vi "SpinnyGlo.vi"() -> ()   [LabVIEW 2014]
uses:
  <vilib>/userdefined/High Color/IMAQdx.ctl
  <vilib>/LabVIEW Interface for Arduino/LabVIEW Interface for Arduino.lvlib
  <vilib>/vision/driver/NI_Vision_Acquisition_Software.lvlib
panel:
  out "Steps per Image":dbl
  out "Total Steps":dbl
  out "Images Acquired":i32
  in  "File Name":string
  in  "Save Location":path
  out "Image":T1(plugin-control)
  out "Degrees per Step":dbl
  out "Degrees per Image":dbl
  in  "Number of Images":dbl
  in  "Camera Name":T2
  out "Steps\nRemaining":u32
  in  "Angular Increment":dbl
  in  "Exit":bool
  in  "Home":bool
  in  "Stop":bool
  in  "MoveToGo":bool
  in  "MoveForGo":bool
  in  "Direction":bool
  out "Current Position":dbl format="%#.2f"
  in  "Move For (+/-360 max)":dbl
  in  "Move To":dbl
  # "CW"
  # "CCW"
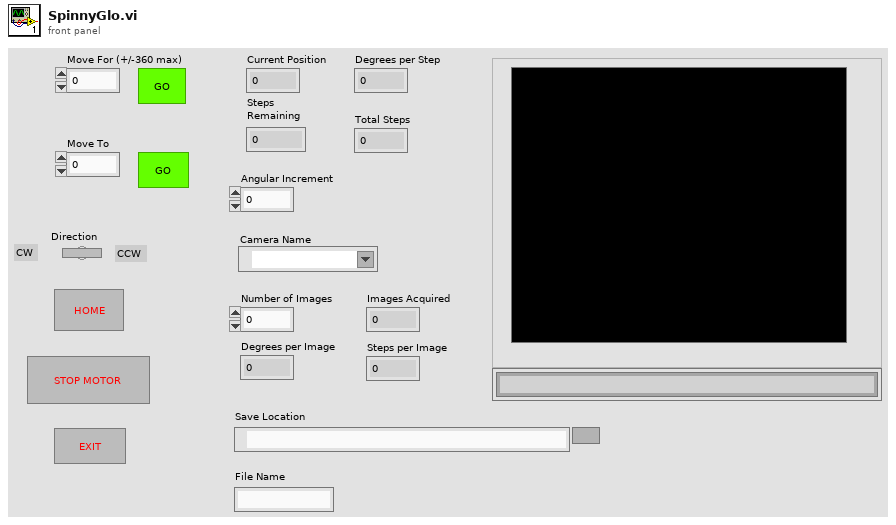
[diagram p1: front panel]
types:
  T1 = typedef "IMAQ Image.ctl" = refnum<image>
  T2 = typedef "IMAQdx.ctl" = refnum<k21>
  T3 = enum16{"Enabled", "Disabled", "Disabled and Grayed Out"}
  T4 = enum8{"Enabled", "Disabled", "Disabled and Grayed Out"}
  T5 = typedef "LabVIEW Interface for Arduino.lvlib/Arduino Resource.ctl" = cluster{"VISA resource":refnum<visa-resource-name>, "Board Type":T6, "Connection Type":enum8{"USB / Serial"}, "Bytes Per Packet (15)":u8}
  T6 = typedef "LabVIEW Interface for Arduino.lvlib/Board Type.ctl" = enum16{"Uno", "Dimuelanove w/Atmega 328", "Mega 2560"}
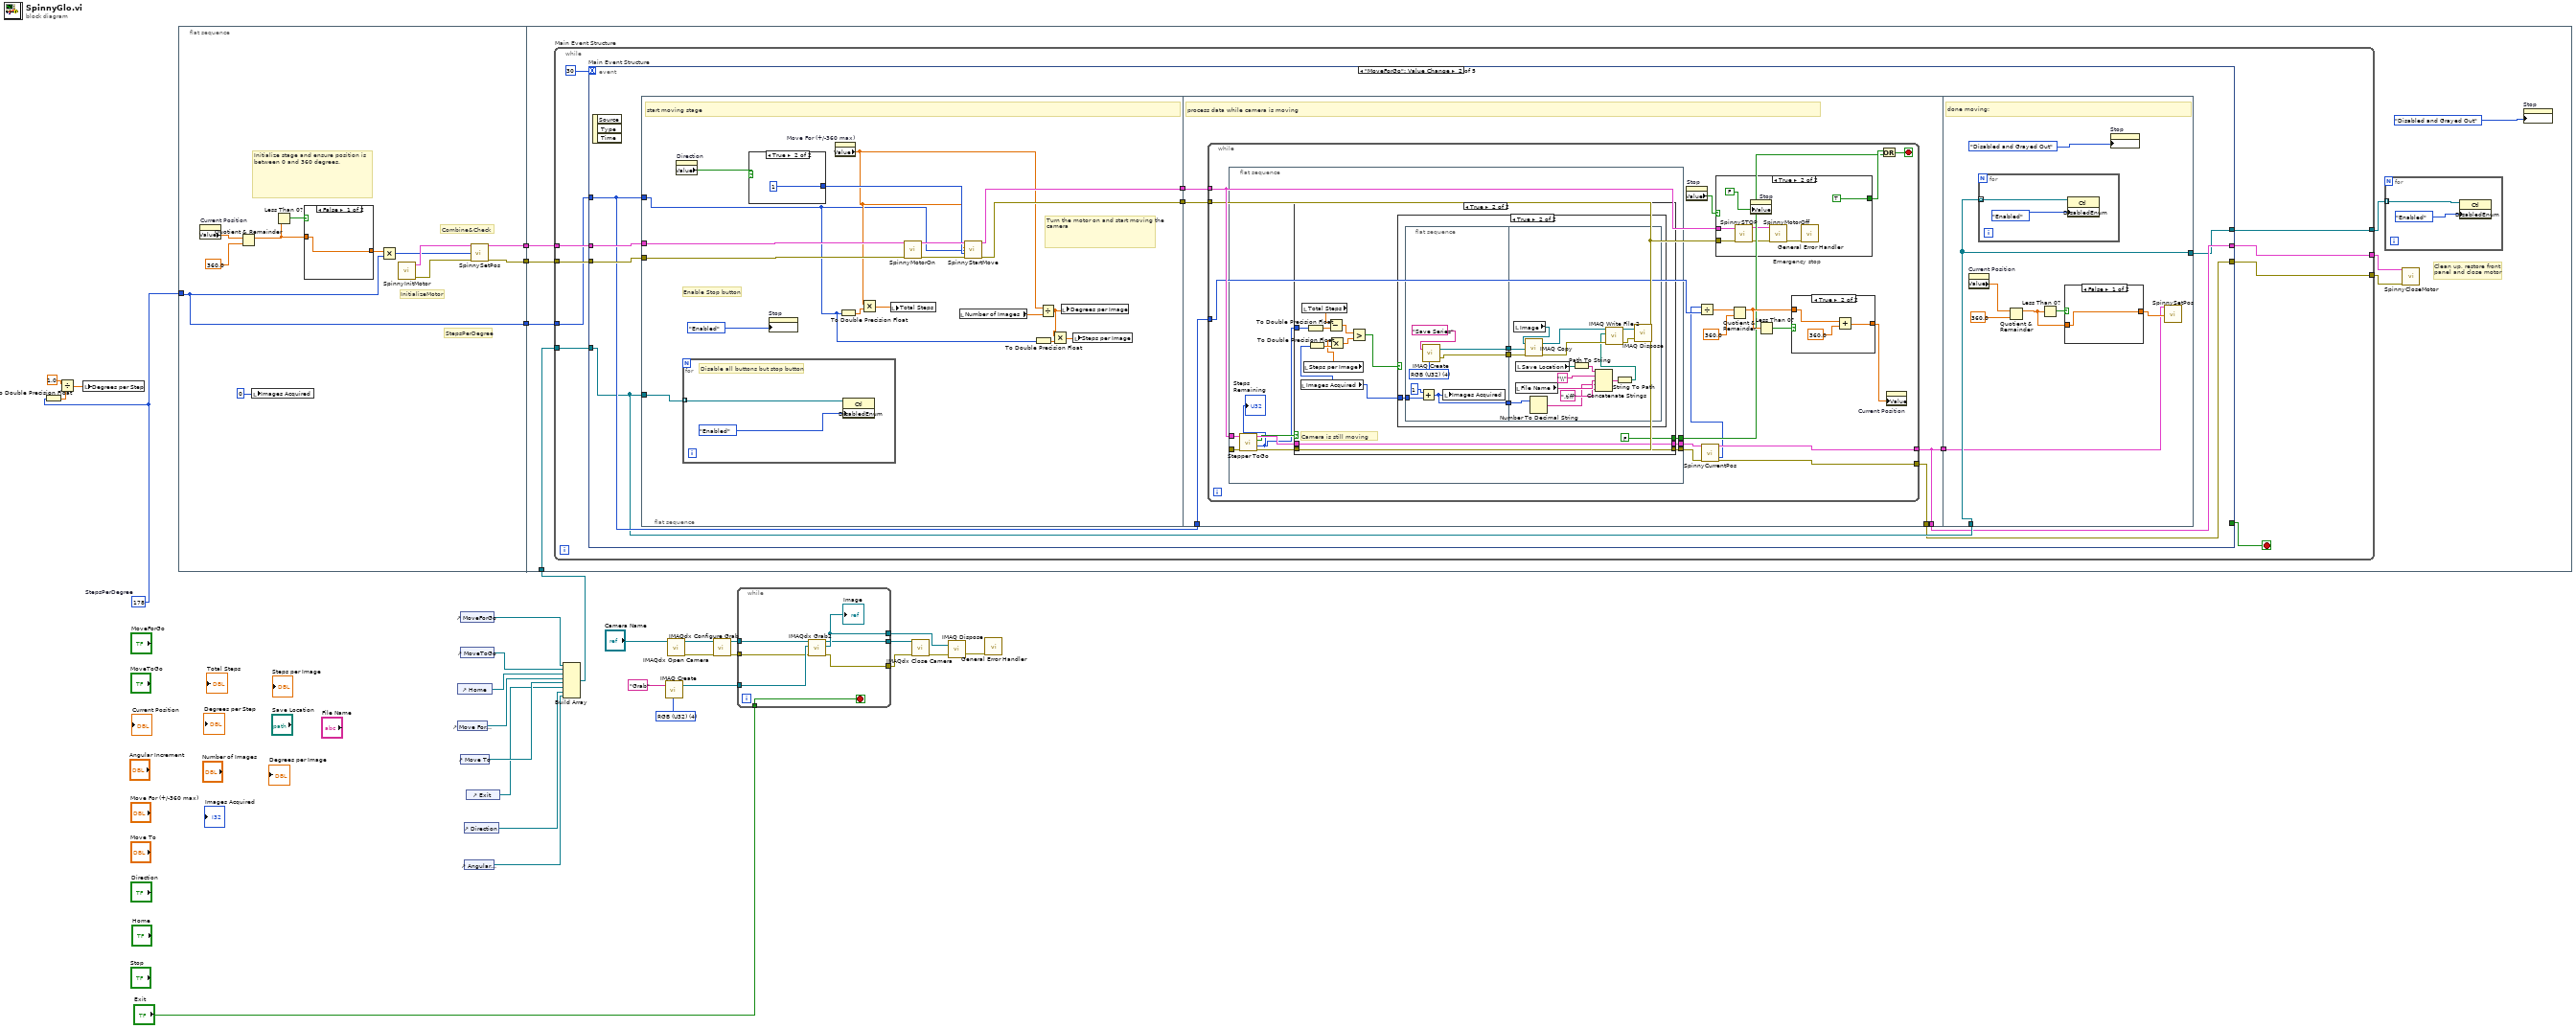
[diagram p0: block diagram]
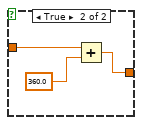
[diagram p2: hidden frame]
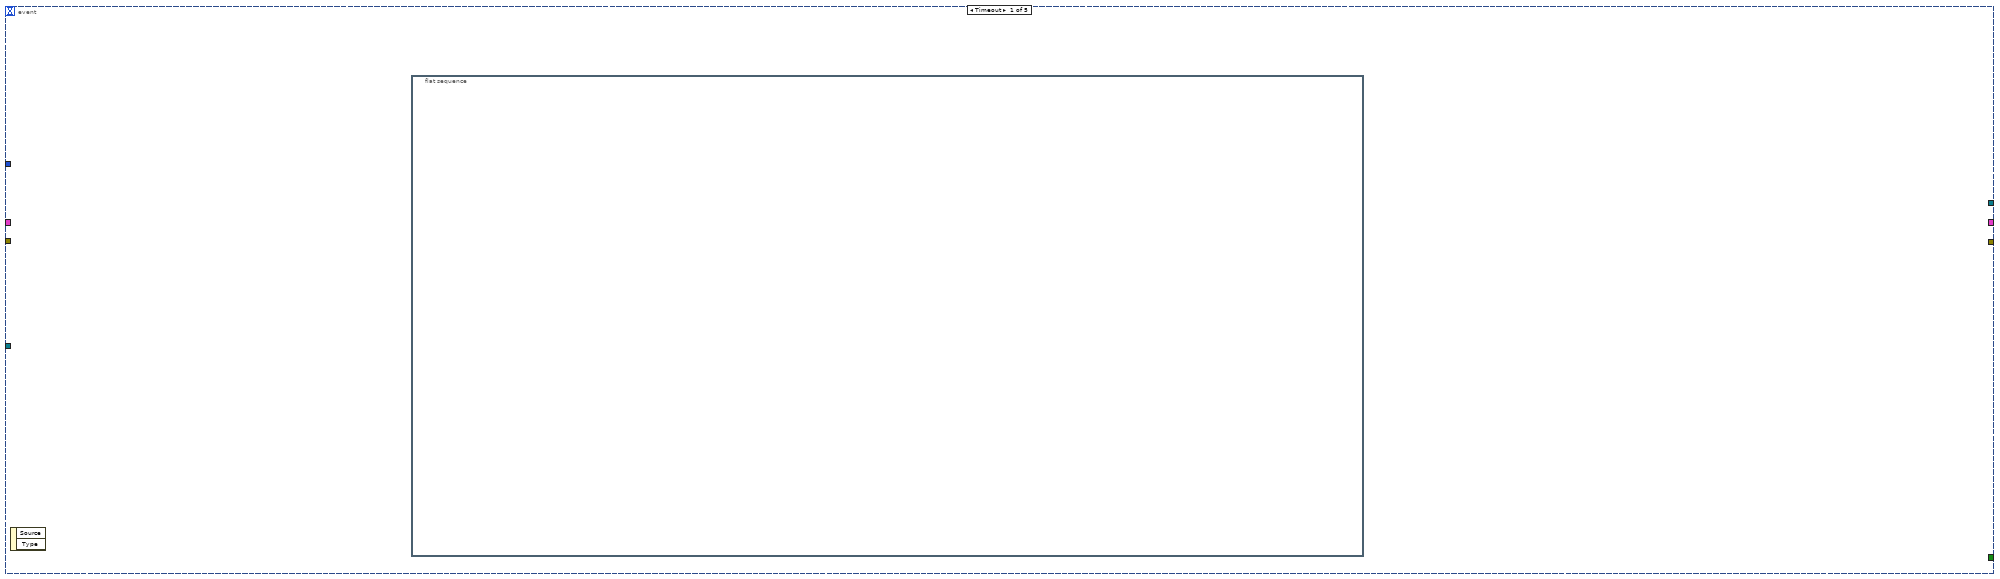
[diagram p3: hidden frame]
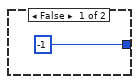
[diagram p4: hidden frame]
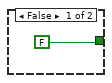
[diagram p6: hidden frame]
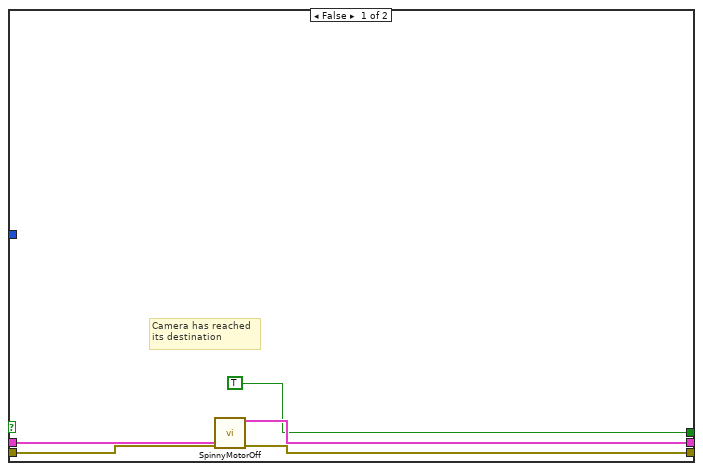
[diagram p7: hidden frame]
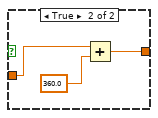
[diagram p9: hidden frame]
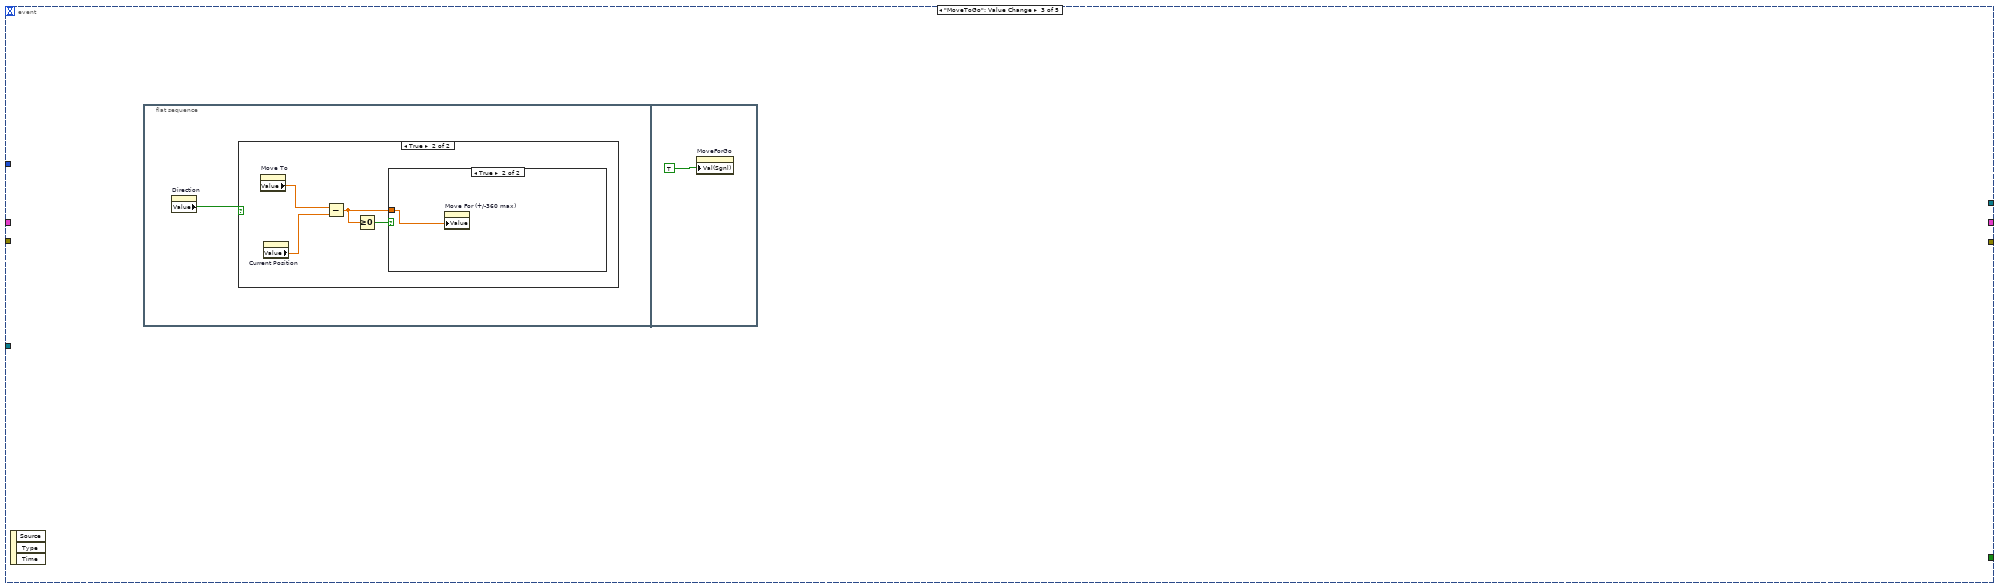
[diagram p10: hidden frame]
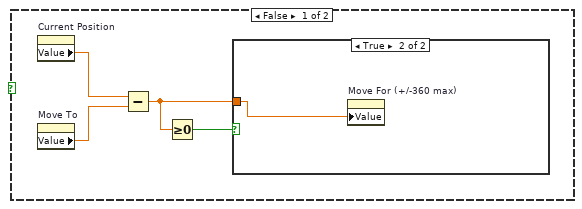
[diagram p11: hidden frame]
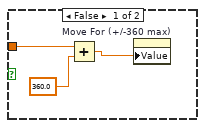
[diagram p12: hidden frame]
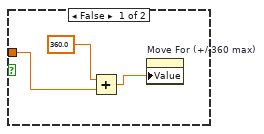
[diagram p13: hidden frame]
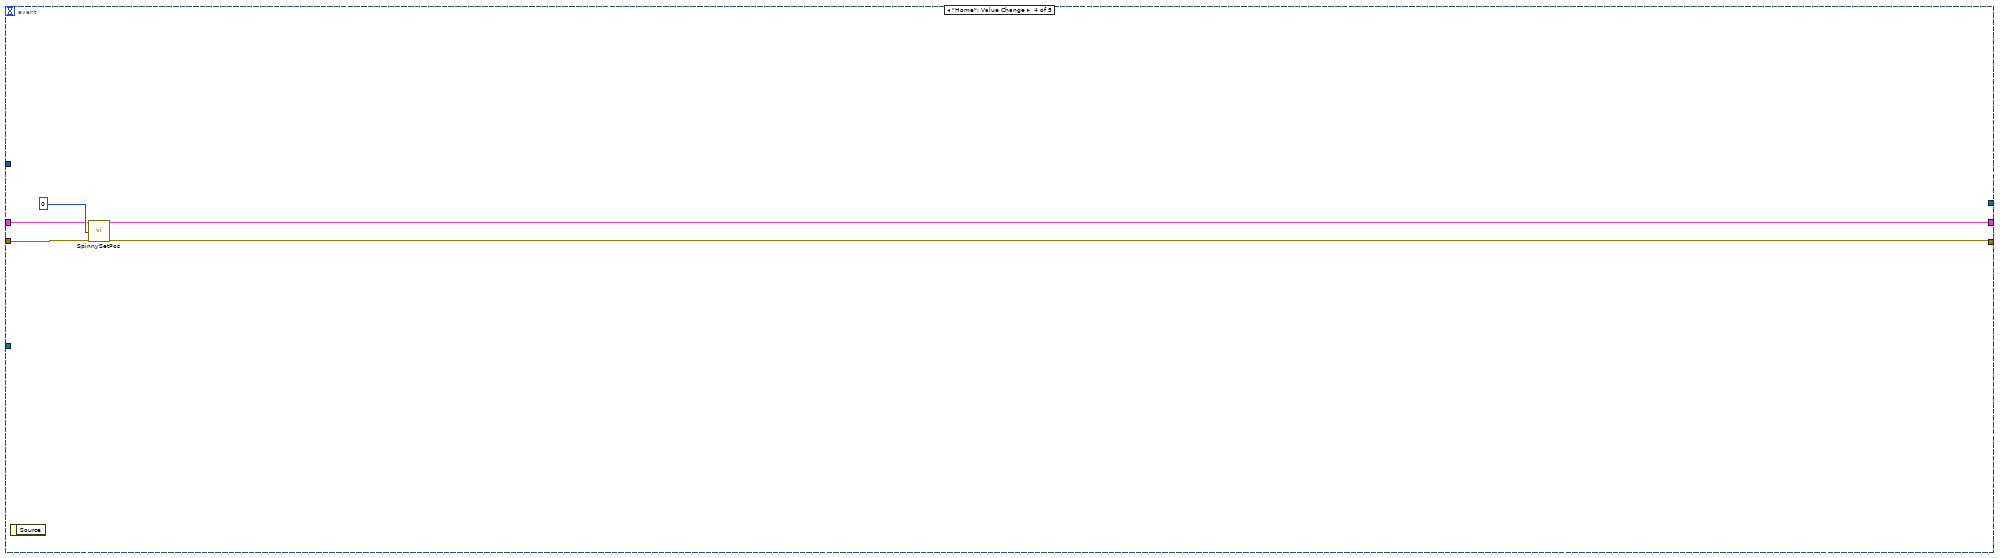
[diagram p14: hidden frame]
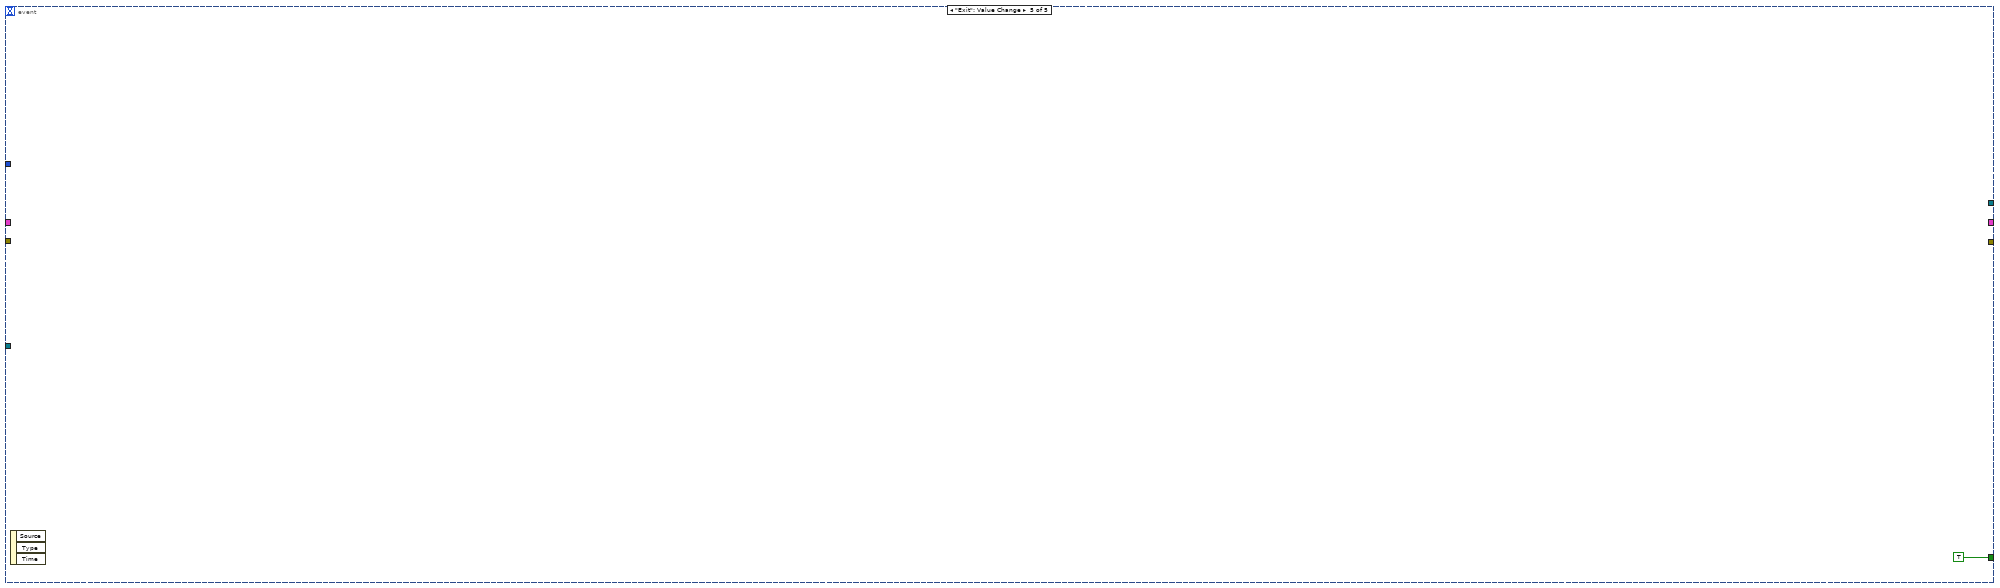
[diagram p15: hidden frame]
diagram:
  w18 = u32 4 items=["Grayscale (U8)", "Grayscale (I16)", "Grayscale (SGL)", "Complex (CSG)", "RGB (U32)", "HSL (U32)", "RGB (U64)", "Grayscale (U16)", ""] ("Image Type")
  w2 = 178  # StepsPerDegree
  n1 = To Double Precision Float(number=w2) -> (double precision float=w5:dbl)
  n2 = Divide(x=1.0, y=w5) -> (x/y=w3:dbl)
  n3 = local write "Degrees per Step"(w3) -> ()
  n4 = flat-sequence {
    tunnel: w2 -> [w32]
    tunnel: [w34] -> w30
    tunnel: [w33] -> w29
    tunnel: [w32] -> w19
    tunnel: w30 -> [w53]
    tunnel: w29 -> [w52]
    tunnel: w20 -> [w54]
    tunnel: w19 -> [w51]
    frame #0 {
      # "StepsPerDegree"
      # "Combine&Check"
      # "InitializeMotor"
      # "Initialize stage and ensure position is between 0 and 360 degrees."
      n5 = property on="Current Position" class="DigNum (strict)"() -> ("Value"=w42:dbl)  [unwired: 2 in, 2 out]
      n6 = Quotient & Remainder(x=w42, y=sgl 360.0) -> (x-y*floor(x/y)=w39:dbl)  [unwired: 1 out]
      n7 = local write "Images Acquired"(0) -> ()
      n8 = Less Than 0?(x=w39) -> (x < 0?=w40:bool)
      n9 = case shown="False" w40 {
        tunnel: w39 -> [w43 w46]
        tunnel: [w43 w44] -> w38
        frame False {
        }
        frame True {
          n10 = Add(x=w46, y=sgl 360.0) -> (x+y=w44:dbl)
        }
      }
      n11 = Multiply(x=w38, y=w32) -> (x*y=w35:i32)
      n12 = call "SpinnyInitMotor.vi"() -> ("error out"=w36:errorcluster, "Arduino Resource Out"=w37:T5)  [unwired: 10 in]
      n13 = call "SpinnySetPos.vi"("Arduino Resource"=w37, "position"=w35, "error in"=w36) -> ("Arduino Resource Out"=w34:T5, "error out"=w33:errorcluster)  [unwired: 15 in]
    }
    frame #1 {
      # "Clean up, restore front\npanel and close motor"
      n14 = while "Main Event Structure" {
        tunnel: w54 -> [w64]
        tunnel: w53 -> [w63]
        tunnel: w52 -> [w62]
        tunnel: w51 -> [w61]
        tunnel: [w60] -> w48
        tunnel: [w59] -> w50
        tunnel: [w58] -> w49
        stop <- w57 stop-if-true
        n15 = event "Main Event Structure" shown="[1] \"MoveForGo\": Value Change" {
          selector: _ -> [_ _ _ _ _]
          dyn-events: _ -> [_ _ _ _ _]
          timeout: 30 -> [_ _ _ _ _]
          tunnel: w64 -> [_ w69 _ _ _]
          tunnel: w63 -> [_ w75 _ w220 _]
          tunnel: w62 -> [_ w74 _ w219 _]
          tunnel: w61 -> [_ w71 _ _ _]
          tunnel: [_ w68 _ w218 _] -> w59
          tunnel: [_ w67 _ w217 _] -> w58
          tunnel: [_ w66 _ _ _] -> w60
          tunnel: [_ _ _ _ TRUE] -> w57
          event Timeout {
            n16 = event-data() -> ()  [unwired: 1 in, 2 out]
            n17 = flat-sequence {
              frame #0 {
              }
            }
          }
          event "MoveForGo": Value Change {
            n18 = event-data() -> ()  [unwired: 1 in, 3 out]
            n19 = flat-sequence {
              tunnel: w69 -> [w93]
              tunnel: w75 -> [w90]
              tunnel: w74 -> [w88]
              tunnel: w71 -> [w79]
              tunnel: [w85] -> w73
              tunnel: [w84] -> w72
              tunnel: w73 -> [w102]
              tunnel: w72 -> [w101]
              tunnel: w71 -> [w100]
              tunnel: [w99] -> w70
              tunnel: [w99] -> w68
              tunnel: [w98] -> w67
              tunnel: w70 -> [w185]
              tunnel: w69 -> [w186]
              tunnel: [w186] -> w66
              frame #0 {
                # "Turn the motor on and start moving the camera"
                # "start moving stage"
                # "Enable Stop button"
                n20 = property on="Direction" class="Bool (strict)"() -> ("Value"=w91:bool)  [unwired: 2 in, 2 out]
                n21 = for {
                  tunnel: w93 -> [w97] mode=indexing
                  # "Disable all buttons but stop button"
                  n22 = property class="Ctl"(reference=w97, "DisabledEnum"=T3."Enabled") -> ()  [unwired: 1 in, 2 out]
                }
                n23 = case shown="True" w91 {
                  tunnel: [-1 1] -> w86
                  frame False {
                  }
                  frame True {
                  }
                }
                n24 = property on="Stop" class="Bool (strict)"("DisabledEnum"=T4."Enabled") -> ()  [unwired: 2 in, 2 out]
                n25 = property on="Move For (+/-360 max)" class="DigNum (strict)"() -> ("Value"=w81:dbl)  [unwired: 2 in, 2 out]
                n26 = To Double Precision Float(number=w79) -> (double precision float=w82:dbl)
                n27 = Multiply(x=w81, y=w82) -> (x*y=w80:dbl)
                n28 = local write "Total Steps"(w80) -> ()
                n29 = call "SpinnyMotorOn.vi"("Arduino Resource"=w90, "error in"=w88) -> ("Arduino Resource Out"=w89:T5, "error out"=w87:errorcluster)  [unwired: 12 in]
                n30 = local read "Number of Images"() -> (w83:dbl)
                n31 = call "SpinnyStartMove.vi"("Arduino Resource"=w89, "Degrees To Move"=w81, "Steps Per Degree"=w79, "Direction"=w86, "error in"=w87) -> ("Arduino Resource Out"=w85:T5, "error out"=w84:errorcluster)  [unwired: 9 in]
                n32 = To Double Precision Float(number=w79) -> (double precision float=w78:dbl)
                n33 = Divide(x=w81, y=w83) -> (x/y=w77:dbl)
                n34 = Multiply(x=w77, y=w78) -> (x*y=w76:dbl)
                n35 = local write "Degrees per Image"(w77) -> ()
                n36 = local write "Steps per Image"(w76) -> ()
              }
              frame #1 {
                # "process data while camera is moving"
                n37 = while {
                  tunnel: w102 -> [w117]
                  tunnel: w101 -> [w116]
                  tunnel: [w115] -> w98
                  tunnel: [w113] -> w99
                  tunnel: w100 -> [w112]
                  stop <- w105 stop-if-true
                  n38 = flat-sequence {
                    tunnel: w116 -> [w140]
                    tunnel: w117 -> [w139]
                    tunnel: [w135] -> w118
                    tunnel: [w134] -> w119
                    tunnel: [w133] -> w106
                    frame #0 {
                      n39 = call <vilib>:"Stepper ToGo.vi"("error in"=w140, "Arduino Resource"=w139) -> ("error out"=w137:errorcluster, "Steps remaining"=w132:u32, "Steps Remaining?"=w136:bool, "Arduino Resource Out"=w138:T5)  [unwired: 6 in]
                      "Steps\nRemaining" <- w132
                      n40 = case shown="True" w136 {
                        tunnel: w138 -> [w145 w157]
                        tunnel: w137 -> [w144 w156]
                        tunnel: [w143 w157] -> w134
                        tunnel: [w142 w156] -> w135
                        tunnel: [TRUE FALSE] -> w133
                        tunnel: w132 -> [_ w154]
                        frame False {
                          # "Camera has reached\nits destination"
                          n41 = call "SpinnyMotorOff.vi"("Arduino Resource"=w145, "error in"=w144) -> ("Arduino Resource Out"=w143:T5, "error out"=w142:errorcluster)  [unwired: 12 in]
                        }
                        frame True {
                          # "Camera is still moving"
                          n42 = local read "Images Acquired"() -> (w148:i32)
                          n43 = local read "Total Steps"() -> (w152:dbl)
                          n44 = local read "Steps per Image"() -> (w147:dbl)
                          n45 = To Double Precision Float(number=w154) -> (double precision float=w153:dbl)
                          n46 = To Double Precision Float(number=w148) -> (double precision float=w149:dbl)
                          n47 = Subtract(x=w152, y=w153) -> (x-y=w151:dbl)
                          n48 = Multiply(x=w147, y=w149) -> (x*y=w146:dbl)
                          n49 = Greater?(x=w151, y=w146) -> (0:w150:bool)
                          n50 = case shown="True" w150 {
                            tunnel: w148 -> [_ w159]
                            frame False {
                            }
                            frame True {
                              n51 = flat-sequence {
                                tunnel: [w166] -> w161
                                tunnel: [w165] -> w160
                                tunnel: w159 -> [w164]
                                tunnel: [w162] -> w158
                                tunnel: w161 -> [w183]
                                tunnel: w160 -> [w179]
                                tunnel: w158 -> [w172]
                                frame #0 {
                                w167 = u16 4 items=["Grayscale (U8)", "Grayscale (I16)", "Grayscale (SGL)", "Complex (CSG)", "RGB (U32)", "HSL (U32)", "RGB (U64)", "Grayscale (U16)", ""]
                                n52 = Add(x=1, y=w164) -> (x+y=w162:i32)
                                n53 = call "IMAQ Create"("Image Name"="Save Series", "Image Type"=w167) -> ("New Image"=w166:T1, "error out"=w165:errorcluster)  [unwired: 3 in]
                                n54 = local write "Images Acquired"(w162) -> ()
                                }
                                frame #1 {
                                n55 = local read "Image"() -> (w184:T1)
                                n56 = local read "File Name"() -> (w174:string)
                                n57 = local read "Save Location"() -> (w176:path)
                                n58 = call "IMAQ Copy"("error in (no error)"=w179, "Image Dst"=w183, "Image Src"=w184) -> ("error out"=w178:errorcluster, "Image Dst Out"=w182:T1)  [unwired: 3 in]
                                n59 = Number To Decimal String(number=w172) -> (decimal integer string=w171:string)  [unwired: 1 in]
                                n60 = Path To String(path=w176) -> (string=w177:string)
                                n61 = Concatenate Strings(w177, "\\", w174, w171, ".tiff") -> (w170:string)
                                n62 = String To Path(string=w170) -> (path=w169:path)
                                n63 = call-poly "IMAQ Write File 2"("error in (no error)"=w178, "File Path"=w169, "Image"=w182) -> ("error out"=w180:errorcluster, "Image Out (duplicate)"=w181:T1)  [unwired: 7 in]
                                n64 = call "IMAQ Dispose"("Image"=w181, "error in (no error)"=w180) -> ()  [unwired: 4 in, 1 out]
                                }
                              }
                            }
                          }
                        }
                      }
                    }
                  }
                  n65 = property on="Stop" class="Bool (strict)"() -> ("Value"=w114:bool)  [unwired: 2 in, 2 out]
                  n66 = call "SpinnyCurrentPos.vi"("Arduino Resource"=w119, "error in"=w118) -> ("Arduino Resource Out"=w113:T5, "position"=w103:i32, "error out"=w115:errorcluster)  [unwired: 15 in]
                  n67 = Divide(x=w103, y=w112) -> (x/y=w111:dbl)
                  n68 = case "Emergency stop" shown="True" w114 {
                    tunnel: w117 -> [_ w131]
                    tunnel: w116 -> [_ w129]
                    tunnel: [FALSE TRUE] -> w107
                    frame False {
                    }
                    frame True {
                      n69 = call "SpinnySTOP.vi"("error in"=w129, "Arduino Resource"=w131) -> ("error out"=w128:errorcluster, "Arduino Resource Out"=w130:T5)  [unwired: 8 in]
                      n70 = property on="Stop" class="Bool (strict)"("Value"=FALSE) -> ()  [unwired: 2 in, 2 out]
                      n71 = call "SpinnyMotorOff.vi"("Arduino Resource"=w130, "error in"=w128) -> ("error out"=w127:errorcluster)  [unwired: 12 in, 1 out]
                      n72 = call <vilib>:"General Error Handler.vi"("error in (no error)"=w127) -> ()  [unwired: 10 in, 5 out]
                    }
                  }
                  n73 = Quotient & Remainder(x=w111, y=sgl 360.0) -> (x-y*floor(x/y)=w109:dbl)  [unwired: 1 out]
                  n74 = Less Than 0?(x=w109) -> (x < 0?=w108:bool)
                  n75 = case shown="True" w108 {
                    tunnel: w109 -> [w120 w122]
                    tunnel: [w120 w121] -> w104
                    frame False {
                    }
                    frame True {
                      n76 = Add(x=w122, y=sgl 360.0) -> (x+y=w121:dbl)
                    }
                  }
                  n77 = Or(x=w107, y=w106) -> (x .or. y?=w105:bool)
                  n78 = property on="Current Position" class="DigNum (strict)"("Value"=w104) -> ()  [unwired: 2 in, 2 out]
                }
              }
              frame #2 {
                # "done moving:"
                n79 = property on="Current Position" class="DigNum (strict)"() -> ("Value"=w191:dbl)  [unwired: 2 in, 2 out]
                n80 = for {
                  tunnel: w186 -> [w197] mode=indexing
                  n81 = property class="Ctl"(reference=w197, "DisabledEnum"=T3."Enabled") -> ()  [unwired: 1 in, 2 out]
                }
                n82 = Quotient & Remainder(x=w191, y=sgl 360.0) -> (x-y*floor(x/y)=w188:dbl)  [unwired: 1 out]
                n83 = Less Than 0?(x=w188) -> (x < 0?=w189:bool)
                n84 = case shown="False" w189 {
                  tunnel: w188 -> [w193 w196]
                  tunnel: [w193 w194] -> w187
                  frame False {
                  }
                  frame True {
                    n85 = Add(x=w196, y=sgl 360.0) -> (x+y=w194:dbl)
                  }
                }
                n86 = property on="Stop" class="Bool (strict)"("DisabledEnum"=T3."Disabled and Grayed Out") -> ()  [unwired: 2 in, 2 out]
                n87 = call "SpinnySetPos.vi"("Arduino Resource"=w185, "position"=w187) -> ()  [unwired: 16 in, 2 out]
              }
            }
          }
          event "MoveToGo": Value Change {
            n88 = event-data() -> ()  [unwired: 1 in, 3 out]
            n89 = flat-sequence {
              frame #0 {
                n90 = property on="Direction" class="Bool (strict)"() -> ("Value"=w199:bool)  [unwired: 2 in, 2 out]
                n91 = case shown="True" w199 {
                  frame False {
                    n92 = property on="Current Position" class="DigNum (strict)"() -> ("Value"=w202:dbl)  [unwired: 2 in, 2 out]
                    n93 = property on="Move To" class="DigNum (strict)"() -> ("Value"=w203:dbl)  [unwired: 2 in, 2 out]
                    n94 = Subtract(x=w202, y=w203) -> (x-y=w200:dbl)
                    n95 = Greater Or Equal To 0?(x=w200) -> (x >= 0?=w201:bool)
                    n96 = case shown="True" w201 {
                      tunnel: w200 -> [w205 w207]
                      frame False {
                        n97 = Add(x=w205, y=sgl 360.0) -> (x+y=w204:dbl)
                        n98 = property on="Move For (+/-360 max)" class="DigNum (strict)"("Value"=w204) -> ()  [unwired: 2 in, 2 out]
                      }
                      frame True {
                        n99 = property on="Move For (+/-360 max)" class="DigNum (strict)"("Value"=w207) -> ()  [unwired: 2 in, 2 out]
                      }
                    }
                  }
                  frame True {
                    n100 = property on="Move To" class="DigNum (strict)"() -> ("Value"=w210:dbl)  [unwired: 2 in, 2 out]
                    n101 = property on="Current Position" class="DigNum (strict)"() -> ("Value"=w211:dbl)  [unwired: 2 in, 2 out]
                    n102 = Subtract(x=w210, y=w211) -> (x-y=w209:dbl)
                    n103 = Greater Or Equal To 0?(x=w209) -> (x >= 0?=w208:bool)
                    n104 = case shown="True" w208 {
                      tunnel: w209 -> [w213 w215]
                      frame False {
                        n105 = Add(x=sgl 360.0, y=w213) -> (x+y=w214:dbl)
                        n106 = property on="Move For (+/-360 max)" class="DigNum (strict)"("Value"=w214) -> ()  [unwired: 2 in, 2 out]
                      }
                      frame True {
                        n107 = property on="Move For (+/-360 max)" class="DigNum (strict)"("Value"=w215) -> ()  [unwired: 2 in, 2 out]
                      }
                    }
                  }
                }
              }
              frame #1 {
                n108 = property on="MoveForGo" class="Bool (strict)"("Val(Sgnl)"=TRUE) -> ()  [unwired: 2 in, 2 out]
              }
            }
          }
          event "Home": Value Change {
            n109 = event-data() -> ()  [unwired: 1 in, 1 out]
            n110 = call "SpinnySetPos.vi"("Arduino Resource"=w220, "position"=0, "error in"=w219) -> ("Arduino Resource Out"=w218:T5, "error out"=w217:errorcluster)  [unwired: 15 in]
          }
          event "Exit": Value Change {
            n111 = event-data() -> ()  [unwired: 1 in, 3 out]
          }
        }
      }
      n112 = for {
        tunnel: w48 -> [w55] mode=indexing
        n113 = property class="Ctl"(reference=w55, "DisabledEnum"=T3."Enabled") -> ()  [unwired: 1 in, 2 out]
      }
      n114 = call "SpinnyCloseMotor.vi"("Arduino Resource"=w50, "error in"=w49) -> ()  [unwired: 18 in]
      n115 = property on="Stop" class="Bool (strict)"("DisabledEnum"=T3."Disabled and Grayed Out") -> ()  [unwired: 2 in, 2 out]
    }
  }
  n116 = control-ref of="Home"() -> (w26:refnum<vi>)
  n117 = control-ref of="Move For (+/-360 max)"() -> (w25:refnum<vi>)
  n118 = control-ref of="MoveForGo"() -> (w28:refnum<vi>)
  n119 = control-ref of="MoveToGo"() -> (w27:refnum<vi>)
  n120 = control-ref of="Move To"() -> (w24:refnum<vi>)
  n121 = control-ref of="Direction"() -> (w22:refnum<vi>)
  n122 = control-ref of="Angular Increment"() -> (w21:refnum<vi>)
  n123 = control-ref of="Exit"() -> (w23:refnum<vi>)
  n124 = Build Array(w28, w27, w26, w25, w24, w23, w22, w21) -> (w20:refnum<vi>[])
  n125 = call "IMAQ Create"("Image Name"="Grab", "Image Type"=w18) -> ("New Image"=w12:T1)  [unwired: 3 in, 1 out]
  n126 = call <vilib>:"IMAQdx Open Camera.vi"("Session In"="Camera Name") -> ("error out"=w15:errorcluster, "Session Out"=w14:T2)  [unwired: 9 in]
  n127 = call <vilib>:"IMAQdx Configure Grab.vi"("error in"=w15, "Session In"=w14) -> ("error out"=w11:errorcluster, "Session Out"=w13:T2)  [unwired: 8 in]
  n128 = while {
    tunnel: w13 -> [w229]
    tunnel: w12 -> [w228]
    tunnel: w11 -> [w227]
    tunnel: [w226] -> w10
    tunnel: [w225] -> w7
    tunnel: [w224] -> w6
    tunnel: "Exit" -> [w223]
    stop <- w223 stop-if-true
    n129 = call <vilib>:"IMAQdx Grab2.vi"("error in"=w227, "Image In"=w228, "Session In"=w229) -> ("error out"=w226:errorcluster, "Image Out"=w225:T1, "Session Out"=w224:T2)  [unwired: 5 in, 1 out]
    "Image" <- w225
  }
  n130 = call <vilib>:"IMAQdx Close Camera.vi"("error in"=w10, "Session In"=w6) -> ("error out"=w9:errorcluster)  [unwired: 9 in]
  n131 = call "IMAQ Dispose"("Image"=w7, "error in (no error)"=w9) -> ("error out"=w8:errorcluster)  [unwired: 4 in]
  n132 = call <vilib>:"General Error Handler.vi"("error in (no error)"=w8) -> ()  [unwired: 10 in, 5 out]
